vi "vfd ramp settings.vi"() -> ()   [LabVIEW 2018]
uses:
  <vilib>/Modbus/subvis/Modbus API/Modbus API.lvclass/Modbus API.ctl
  <vilib>/Modbus/subvis/Transmission Data Unit (ADU)/Transmission Data Unit/Transmission Data Unit.lvclass/Transmission Data Unit.ctl
  <vilib>/Modbus/master/Data Access/Unit ID/Set Unit ID Property.vi
  <vilib>/Modbus/subvis/Transmission Data Unit (ADU)/Transmission Data Unit/Data Access/Unit ID/Write Unit ID.vi
  <vilib>/Modbus/subvis/Modbus API/Read Transmission Data Unit.vi
  <vilib>/Modbus/subvis/Modbus API/Write Transmission Data Unit.vi
  <vilib>/Modbus/master/Modbus Master.lvclass
  C:/Program Files (x86)/National Instruments/LabVIEW 2018/vi.lib/Modbus/subvis/Modbus API/Modbus API.lvclass
  <vilib>/Modbus/master/Create Master Instance (TCP).vi
  <vilib>/Modbus/subvis/Transmission Data Unit (ADU)/Transmission Data Unit/Transmission Data Unit.lvclass
panel:
  out "register values":u16[][](array[numeric])
  in  "OverSpeed Threshold":u16
  in  "Deacceleration Rate 1":dbl
  in  "Acceleration Rate 1":dbl
  in  "Maximum Reference Clamp":dbl
  in  "Minimum Reference Clamp":dbl
  in  "Set Speed":dbl
  out "Array":dbl[](array[numeric])
  in  "stop":bool
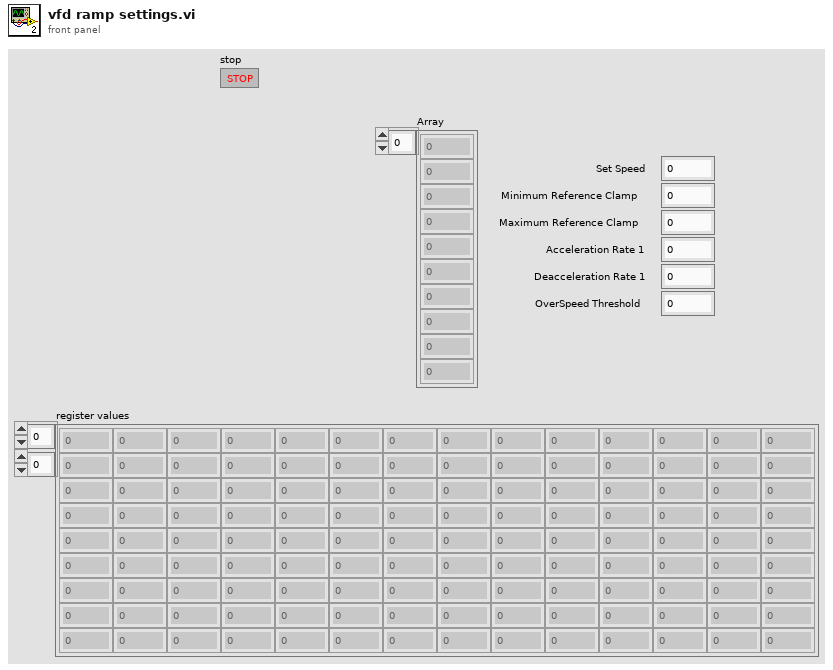
[diagram p1: front panel]
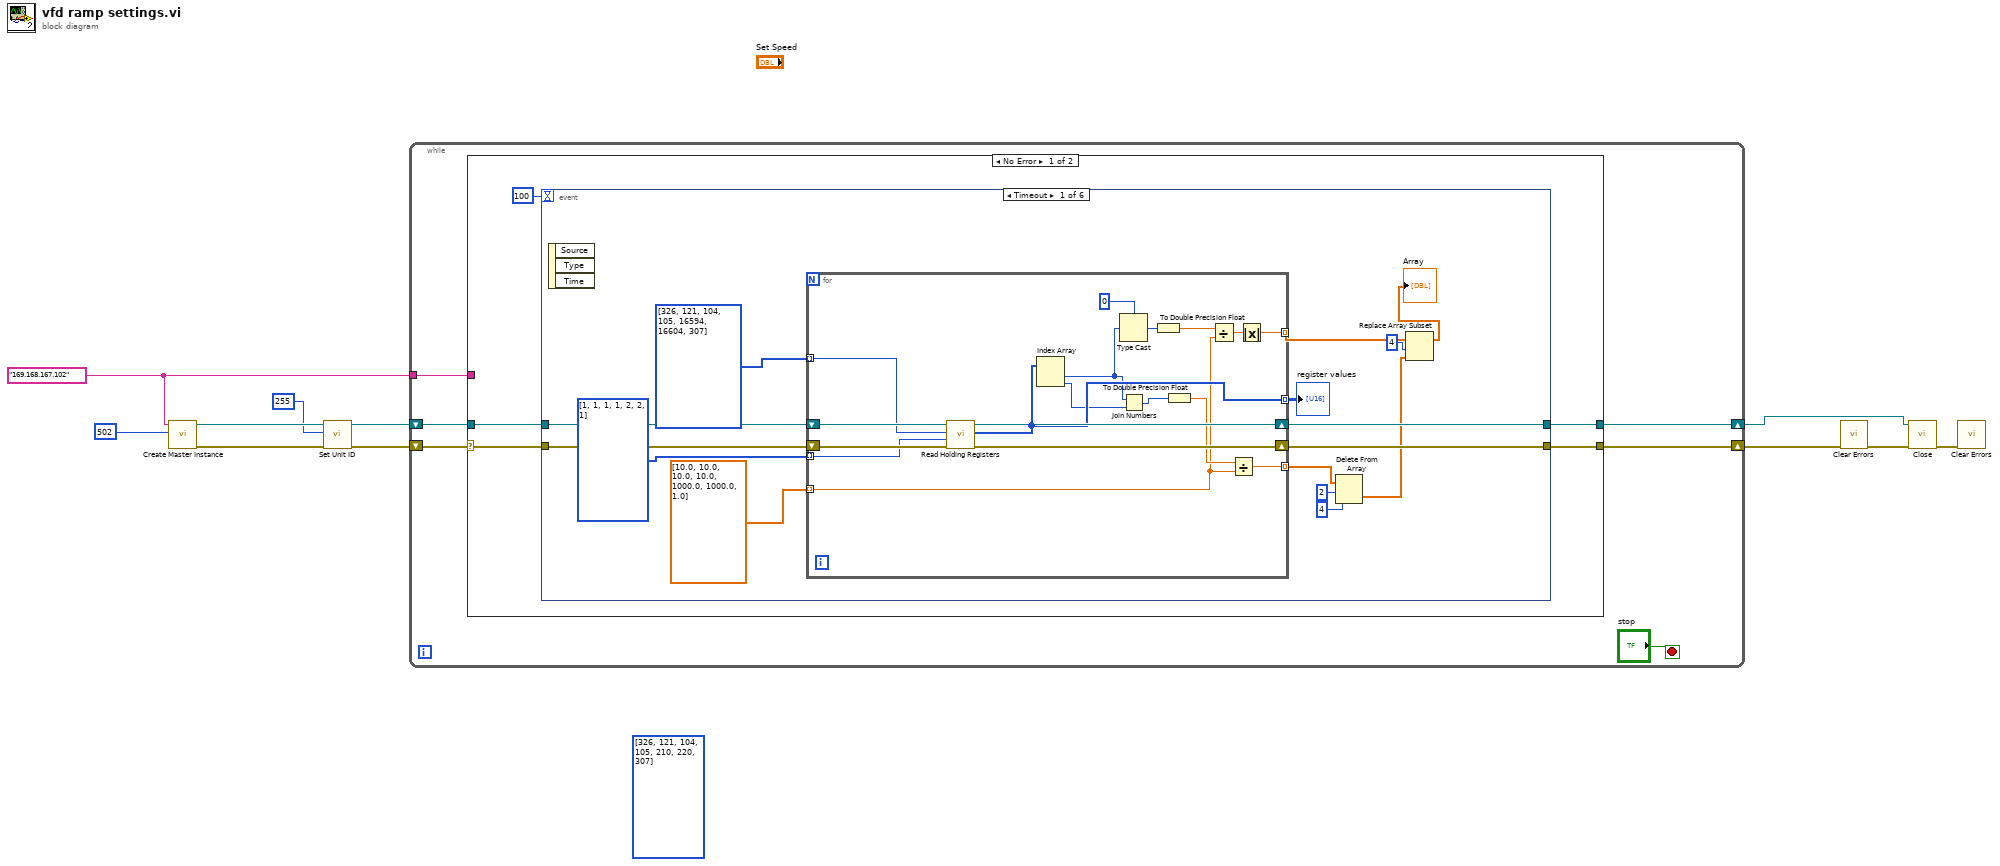
[diagram p0: block diagram]
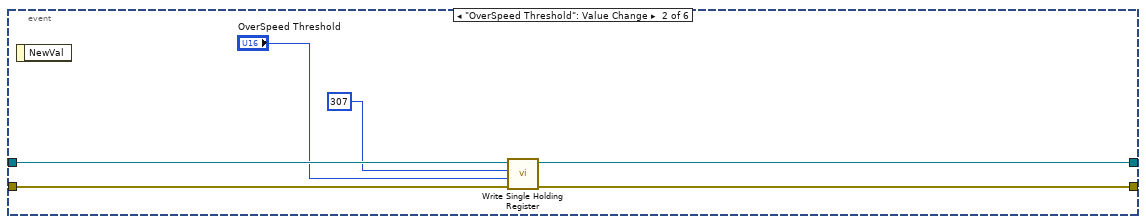
[diagram p2: hidden frame]
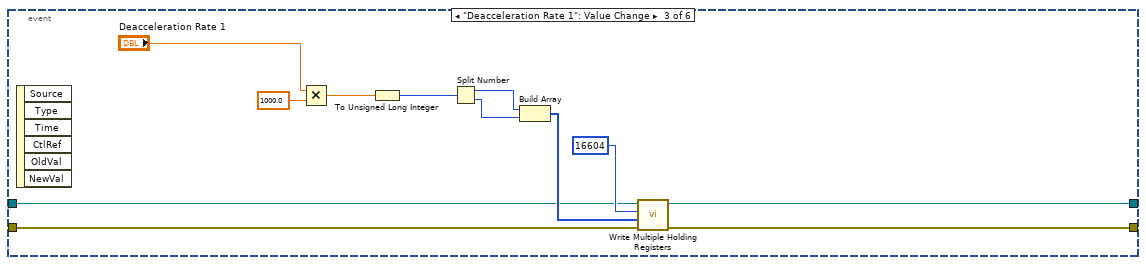
[diagram p3: hidden frame]
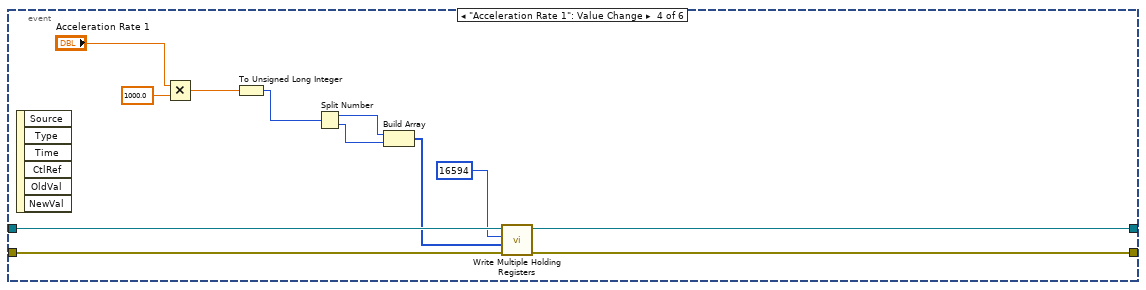
[diagram p4: hidden frame]
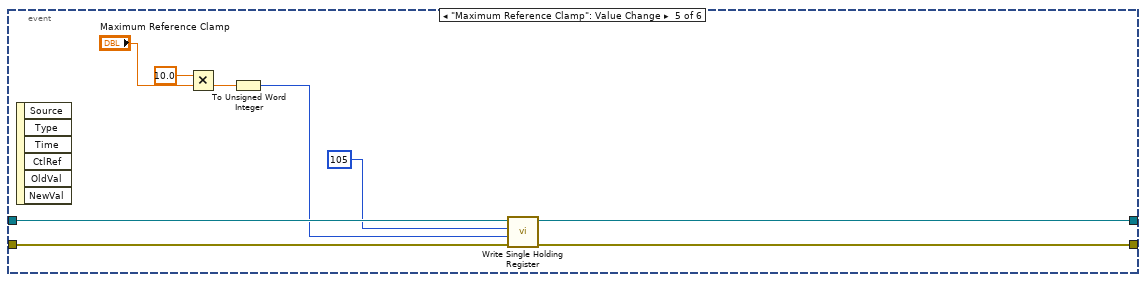
[diagram p5: hidden frame]
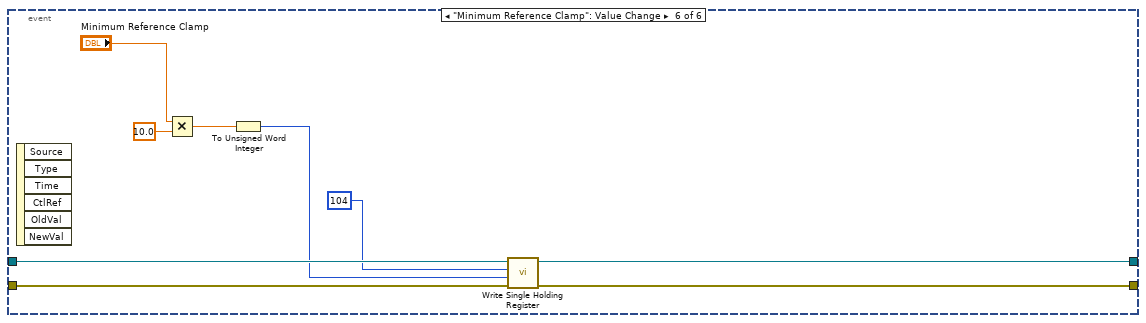
[diagram p6: hidden frame]
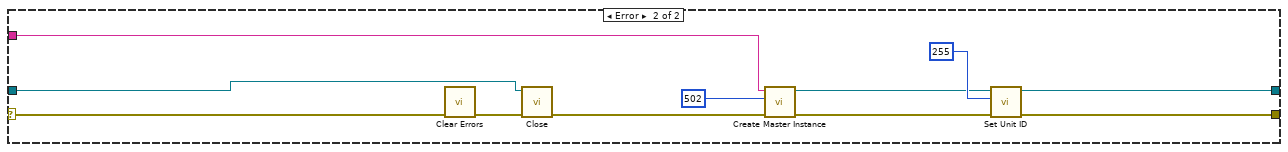
[diagram p7: hidden frame]
diagram:
  (unwired) u16[] [326, 121, 104, 105, 210, 220, 307] ("starting address")
  w1 = "169.168.167.102" ("address")
  n1 = call-poly <vilib>:"Create Master Instance.vi"("port (502)"=u16 502, "address"=w1) -> ("error out"=w10:errorcluster, "TCP master instance"=w9:refnum<class "Modbus Master.lvclass">)  [unwired: 8 in]
  n2 = call <vilib>:"Set Unit ID.vi"("error in (no error)"=w10, "unit ID"=u8 255, "Modbus master in"=w9) -> ("error out"=w6:errorcluster, "Modbus master out"=w7:refnum<class "Modbus Master.lvclass">)  [unwired: 7 in]
  n3 = while {
    shift-right: [w17] -> w4
    shift-left: w6 -> [w16]
    shift-right: [w13] -> w3
    shift-left: w7 -> [w15]
    tunnel: w1 -> [w12]
    stop <- "stop" stop-if-true
    n4 = case shown="No Error" w16 {
      selector: w16 -> [w20 w114]
      tunnel: [w19 w107] -> w17
      tunnel: w15 -> [w21 w105]
      tunnel: [w18 w106] -> w13
      tunnel: w12 -> [_ w104]
      frame No Error {
        n5 = event shown="[0] Timeout" {
          selector: _ -> [_ _ _ _ _ _]
          dyn-events: _ -> [_ _ _ _ _ _]
          timeout: 100 -> [_ _ _ _ _ _]
          tunnel: w21 -> [w36 w61 w63 w82 w94 w103]
          tunnel: w20 -> [w37 w60 w66 w80 w93 w102]
          tunnel: [w34 w57 w65 w79 w91 w100] -> w19
          tunnel: [w33 w56 w64 w81 w90 w99] -> w18
          event Timeout {
            n6 = event-data() -> ()  [unwired: 1 in, 3 out]
            n7 = for {
              tunnel: u16[] [326, 121, 104, 105, 16594, 16604, 307] ("starting address") -> [w53] mode=indexing
              shift-right: [w52] -> w34
              shift-left: w37 -> [w55]
              shift-right: [w51] -> w33
              shift-left: w36 -> [w54]
              tunnel: [w46] -> w26 mode=indexing
              tunnel: dbl[] [10.0, 10.0, 10.0, 10.0, 1000.0, 1000.0, 1.0] -> [w39] mode=indexing
              tunnel: u16[] [1, 1, 1, 1, 2, 2, 1] ("starting address") -> [w45] mode=indexing
              tunnel: [w44] -> w30 mode=indexing
              tunnel: [w38] -> w29 mode=indexing
              n8 = call-dynamic "Read Holding Registers.vi"("error in (no error)"=w55, "number of holding registers"=w45, "starting address"=w53, "Modbus master in"=w54) -> ("error out"=w52:errorcluster, "register values"=w44:u16[], "Modbus master out"=w51:refnum<class "Modbus Master.lvclass">)  [unwired: 5 in]
              n9 = Index Array(array=w44) -> (element #1=w43:u16, element #2=w42:u16)  [unwired: 2 in]
              n10 = Type Cast(type=i16 0, x=w43) -> (*(type *) &x=w50:i16)
              n11 = Join Numbers(hi=w43, lo=w42) -> ((hi.lo)=w41:u32)
              n12 = To Double Precision Float(number=w50) -> (double precision float=w49:dbl)
              n13 = To Double Precision Float(number=w41) -> (double precision float=w40:dbl)
              n14 = Divide(x=w49, y=w39) -> (x/y=w48:dbl)
              n15 = Divide(x=w40, y=w39) -> (x/y=w38:dbl)
              n16 = Absolute Value(x=w48) -> (abs(x)=w46:dbl)
            }
            "register values" <- w30
            n17 = Delete From Array(array=w29, length=2, index=4) -> (deleted portion=w25:dbl[])  [unwired: 1 out]
            n18 = Replace Array Subset(array=w26, new element=w25, index=4) -> (→"Array":dbl[])
          }
          event "OverSpeed Threshold": Value Change {
            n19 = event-data() -> ()  [unwired: 1 in, 1 out]
            n20 = call-dynamic "Write Single Holding Register.vi"("error in (no error)"=w60, "holding register value"="OverSpeed Threshold", "address"=u16 307, "Modbus master in"=w61) -> ("error out"=w57:errorcluster, "Modbus master out"=w56:refnum<class "Modbus Master.lvclass">)  [unwired: 6 in]
          }
          event "Deacceleration Rate 1": Value Change {
            n21 = event-data() -> ()  [unwired: 1 in, 6 out]
            n22 = Multiply(x="Deacceleration Rate 1", y=1000.0) -> (x*y=w73:dbl)
            n23 = To Unsigned Long Integer(number=w73) -> (unsigned 32bit integer=w72:u32)
            n24 = Split Number(x=w72) -> (hi(x)=w71:u16, lo(x)=w70:u16)
            n25 = Build Array(w71, w70) -> (w69:u16[])
            n26 = call-dynamic "Write Multiple Holding Registers.vi"("error in (no error)"=w66, "holding register values"=w69, "starting address"=u16 16604, "Modbus master in"=w63) -> ("error out"=w65:errorcluster, "Modbus master out"=w64:refnum<class "Modbus Master.lvclass">)  [unwired: 6 in]
          }
          event "Acceleration Rate 1": Value Change {
            n27 = event-data() -> ()  [unwired: 1 in, 6 out]
            n28 = Multiply(x="Acceleration Rate 1", y=1000.0) -> (x*y=w83:dbl)
            n29 = To Unsigned Long Integer(number=w83) -> (unsigned 32bit integer=w78:u32)
            n30 = Split Number(x=w78) -> (hi(x)=w77:u16, lo(x)=w76:u16)
            n31 = Build Array(w77, w76) -> (w75:u16[])
            n32 = call-dynamic "Write Multiple Holding Registers.vi"("error in (no error)"=w80, "holding register values"=w75, "starting address"=u16 16594, "Modbus master in"=w82) -> ("error out"=w79:errorcluster, "Modbus master out"=w81:refnum<class "Modbus Master.lvclass">)  [unwired: 6 in]
          }
          event "Maximum Reference Clamp": Value Change {
            n33 = event-data() -> ()  [unwired: 1 in, 6 out]
            n34 = Multiply(x=10.0, y="Maximum Reference Clamp") -> (x*y=w87:dbl)
            n35 = To Unsigned Word Integer(number=w87) -> (unsigned 16bit integer=w89:u16)
            n36 = call-dynamic "Write Single Holding Register.vi"("error in (no error)"=w93, "holding register value"=w89, "address"=u16 105, "Modbus master in"=w94) -> ("error out"=w91:errorcluster, "Modbus master out"=w90:refnum<class "Modbus Master.lvclass">)  [unwired: 6 in]
          }
          event "Minimum Reference Clamp": Value Change {
            n37 = event-data() -> ()  [unwired: 1 in, 6 out]
            n38 = Multiply(x="Minimum Reference Clamp", y=10.0) -> (x*y=w97:dbl)
            n39 = To Unsigned Word Integer(number=w97) -> (unsigned 16bit integer=w96:u16)
            n40 = call-dynamic "Write Single Holding Register.vi"("error in (no error)"=w102, "holding register value"=w96, "address"=u16 104, "Modbus master in"=w103) -> ("error out"=w100:errorcluster, "Modbus master out"=w99:refnum<class "Modbus Master.lvclass">)  [unwired: 6 in]
          }
        }
      }
      frame Error {
        n41 = call <vilib>:"Clear Errors.vi"("error in (no error)"=w114) -> ("error out"=w113:errorcluster)  [unwired: 5 in, 1 out]
        n42 = call-dynamic "Close.vi"("error in (no error)"=w113, "Modbus master in"=w105) -> ("error out"=w111:errorcluster)  [unwired: 9 in]
        n43 = call-poly <vilib>:"Create Master Instance.vi"("error in (no error)"=w111, "port (502)"=u16 502, "address"=w104) -> ("error out"=w109:errorcluster, "TCP master instance"=w108:refnum<class "Modbus Master.lvclass">)  [unwired: 7 in]
        n44 = call <vilib>:"Set Unit ID.vi"("error in (no error)"=w109, "unit ID"=u8 255, "Modbus master in"=w108) -> ("error out"=w107:errorcluster, "Modbus master out"=w106:refnum<class "Modbus Master.lvclass">)  [unwired: 7 in]
      }
    }
  }
  n45 = call <vilib>:"Clear Errors.vi"("error in (no error)"=w4) -> ("error out"=w5:errorcluster)  [unwired: 5 in, 1 out]
  n46 = call-dynamic "Close.vi"("error in (no error)"=w5, "Modbus master in"=w3) -> ("error out"=w2:errorcluster)  [unwired: 9 in]
  n47 = call <vilib>:"Clear Errors.vi"("error in (no error)"=w2) -> ()  [unwired: 5 in, 2 out]
